vi "Destroy References.vi"(7 "error in":errorcluster, 10 "Queue References":T1) -> (0 "error out":errorcluster)   [LabVIEW 2014, in "QueueMaintenance.lvlib"]
doc: "Queue Reference:\n\nDefines name queue references for each of the queued state machines. This includes a custom control for both the queue data type (cluster) and a custer of all the queue refnums."
uses:
  QueueMaintenance.lvlib
  TypeDef/QSMRef_ALL.ctl
  Queue_TESTGUIUPDATE/Controls/QSM_Reference.ctl
  Queue_TESTGUIUPDATE/Controls/QSM_DataType.ctl
  Queue_TESTGUIUPDATE/Controls/QSM_RunStates.ctl
  Queue_TEST/Controls/QSM_Reference.ctl
  Queue_TEST/Controls/QSM_DataType.ctl
  Queue_TEST/Controls/QSM_RunStates.ctl
  Queue_TEST/TestQSM.lvlib
  Queue_TESTGUIUPDATE/GUIUpdateQSM.lvlib
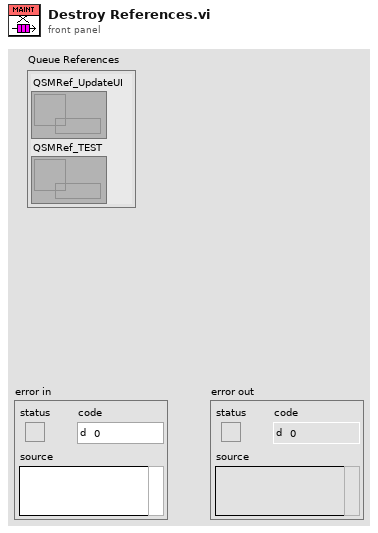
[diagram p1: front panel]
types:
  T1 = typedef "QueueMaintenance.lvlib/QSMRef_ALL.ctl" = cluster{"QSMRef_UpdateUI":T2, "QSMRef_TEST":T3}
  T2 = typedef "GUIUpdateQSM.lvlib/QSM_Reference.ctl" = refnum<queue>
  T3 = typedef "TestQSM.lvlib/QSM_Reference.ctl" = refnum<queue>
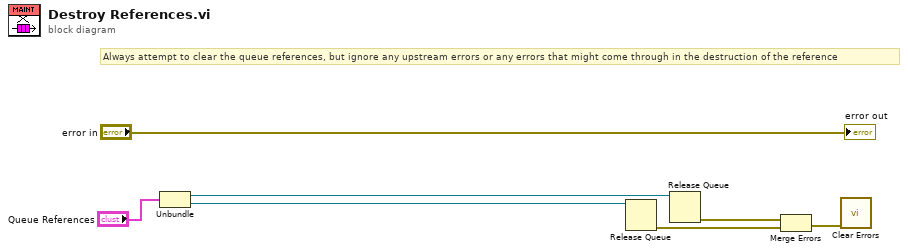
[diagram p0: block diagram]
diagram:
  # "Always attempt to clear the queue references, but ignore any upstream errors or any errors that might come through in the destruction of the reference"
  n1 = Unbundle("Queue References") -> ("QSMRef_UpdateUI"=w5:T2, "QSMRef_TEST"=w6:T3)
  n2 = Release Queue(queue=w6) -> (error out=w3:errorcluster)  [unwired: 2 in, 2 out]
  n3 = Release Queue(queue=w5) -> (error out=w4:errorcluster)  [unwired: 2 in, 2 out]
  n4 = Merge Errors(w4, w3) -> (w1:errorcluster)
  n5 = call <vilib>:"Clear Errors.vi"("error in (no error)"=w1) -> ()  [unwired: 5 in, 2 out]
  "error out" <- "error in"
